vi "Lin_pot_voltage_to_mm_Right.vi"(2 "Offset":dbl, 3 "Gradient":dbl, 4 "LinPot Voltage":dbl) -> (0 "LinPot mm (center to finger)":dbl, 1 "LinPot mm (finger to finger)":dbl)   [LabVIEW 2019]
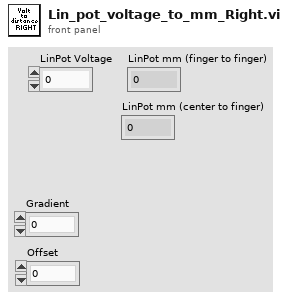
[diagram p1: front panel]
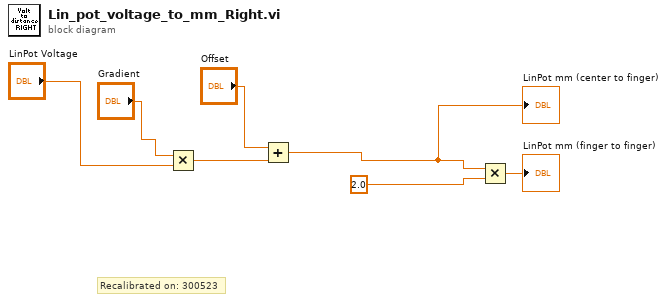
[diagram p0: block diagram]
diagram:
  # "Recalibrated on: 300523"
  n1 = Multiply(x="Gradient", y="LinPot Voltage") -> (x*y=w4:dbl)
  n2 = Add(x="Offset", y=w4) -> (x+y=w3:dbl)
  "LinPot mm (center to finger)" <- w3
  n3 = Multiply(x=w3, y=2.0) -> (x*y=→"LinPot mm (finger to finger)":dbl)
